vi "LVClass_ModalCoef GetLegendrePrefs.vi"(0 "ModalCoef in":refnum<class "ModalCoef.lvclass">, 11 "error in (no error)":errorcluster) -> (4 "ModalCoef out":refnum<class "ModalCoef.lvclass">, 6 "LegendreModalPrefs":T1={"Number of coefficients"=32, "Filtered coefficients"=[], "RectangularProjectionPupilDimensions"={"Pupil center_sspp"={"X"=0.0, "Y"=0.0}, "Pupil halfsize_sspp"={"X"=0.0, "Y"=0.0}}}, 15 "error out":errorcluster)   [LabVIEW 2020, in "ModalCoef.lvclass"]
doc: "Get preferences for phase reconstruction from Legendre decomposition.\n\n--------------------------------------------------------------------------------\n\n<B>ComputePhaseSetIn </B> : ComputePhaseSet object.\n<B>ComputePhaseSetOut </B> : ComputePhaseSet object.\n<B>nb_coeffs_total </B> : Number of the Legendre coefficients used in the polynomial base.\n<B>nb_coeffs_to_filter </B> : Number of the Legendre coefficients to filter in the polynomial base.\n<B>coeffs_to_filter </B> : Indices of the Legendre coefficients to filter in the polynomial base.\n<B>projection_pupil_center </B> : Center of the projection pupil,in number of subpupils.\n<B>projection_pupil_halfsize </B> : Projection pupil half-size, in number of subpupils.\n<B>ErrorIn </B> : Error\n<B>ErrorOut </B> : Error\n\n--------------------------------------------------------------------------------"
uses:
  ModalCoef.lvclass
  LegendreModalPrefs.ctl
  LegendreProjectionPupilSetup.ctl
  Point2Df.ctl
  ModalCoef.lvclass/ModalCoef.ctl
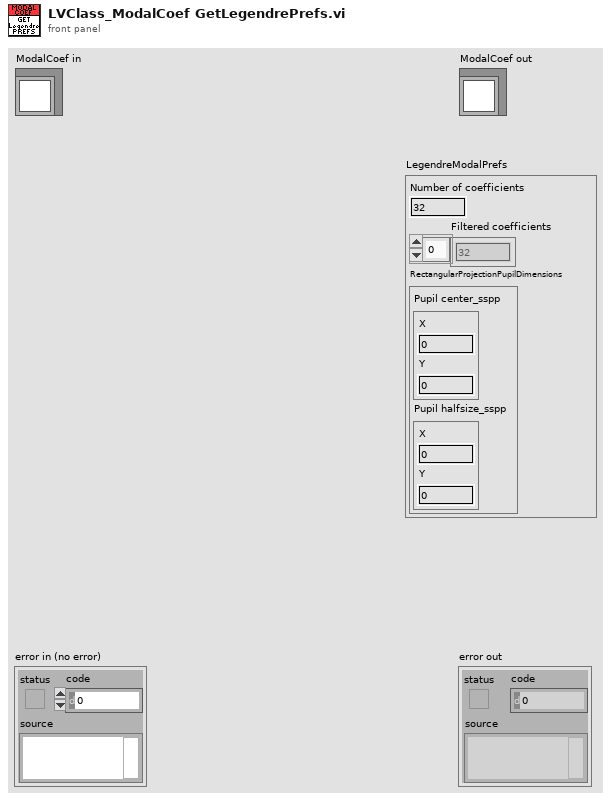
[diagram p1: front panel]
types:
  T1 = typedef "LegendreModalPrefs.ctl" = cluster{"Number of coefficients":u32, "Filtered coefficients":u32[], "RectangularProjectionPupilDimensions":T2}
  T2 = typedef "LegendreProjectionPupilSetup.ctl" = cluster{"Pupil center_sspp":T3, "Pupil halfsize_sspp":T3}
  T3 = typedef "Point2Df.ctl" = cluster{"X":sgl, "Y":sgl}
  T4 = cluster{"Number of coefficients":u32, "Filtered coefficients":u32[], "RectangularProjectionPupilDimensions":T2}
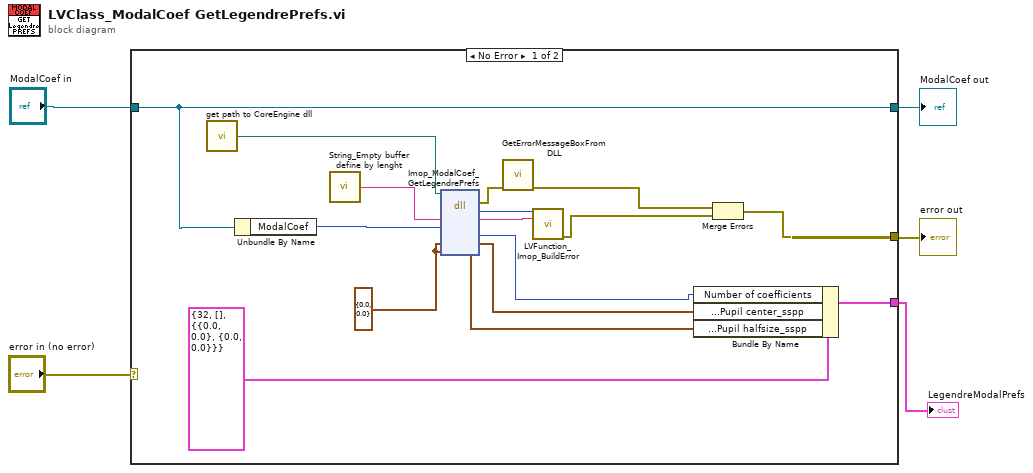
[diagram p0: block diagram]
diagram:
  n1 = case shown="No Error" "error in (no error)" {
    selector: "error in (no error)" -> [_ w23]
    tunnel: [w6 w23] -> w2
    tunnel: [w10 w22] -> w4
    tunnel: "ModalCoef in" -> [w10 w22]
    tunnel: [w16 _] -> w1
    frame No Error {
      w13 = T3 {"X"=0.0, "Y"=0.0} ("RectangularProjectionPupilDimensions.Pupil center_sspp")
      n2 = call "get path to CoreEngine dll.vi"() -> ("path to c_interface_vc100.dll"=w18:path)  [unwired: 12 in, 3 out]
      n3 = Unbundle By Name(w10) -> ("ModalCoef"=w9:i32)
      n4 = call "String_Empty buffer define by lenght.vi"() -> ("Empty buffer"=w19:string)  [unwired: 1 in]
      n5 = dll-call lib="D:/2_trunk/Soft_haso/ImOpCoreEngine4_LV2011/DLLs/ImopEngine4_vc100.dll" fn="Imop_ModalCoef_GetLegendrePrefs"(path in=w18, "message"=w19, "objet"=w9, "projection_pupil_center"=w13, "projection_pupil_size"=w13) -> (error out=w17:errorcluster, "return type"=w21:i32, "message"=w20:string, "numberOfCoefficient"=w11:u32, "projection_pupil_center"=w14:T3, "projection_pupil_size"=w12:T3)  [unwired: 4 in, 1 out]
      n6 = call "GetErrorMessageBoxFromDLL.vi"("error IN"=w17) -> ("error OUT"=w8:errorcluster)  [unwired: 10 in]
      n7 = call "LVFunction_Imop_BuildError.vi"("code"=w21, "String to Prepend to source (\"\")"=w20) -> ("error out"=w7:errorcluster)  [unwired: 13 in]
      n8 = Bundle By Name(cluster=T4 {"Number of coefficients"=32, "Filtered coefficients"=[], "RectangularProjectionPupilDimensions"={"Pupil center_sspp"={"X"=0.0, "Y"=0.0}, "Pupil halfsize_sspp"={"X"=0.0, "Y"=0.0}}} ("LegendreModalPrefs"), "Number of coefficients"=w11, "RectangularProjectionPupilDimensions.Pupil center_sspp"=w14, "RectangularProjectionPupilDimensions.Pupil halfsize_sspp"=w12) -> (w16:T4)
      n9 = Merge Errors(w8, w7) -> (w6:errorcluster)
    }
    frame Error {
    }
  }
  "error out" <- w2
  "ModalCoef out" <- w4
  "LegendreModalPrefs" <- w1
